vi "main.vi"() -> ()   [LabVIEW 2021]
uses:
  <vilib>/MakerHub/LINX/Private/Device/Type Defs/Stimulus Pulse.ctl
  <vilib>/MakerHub/LINX/Public/Utilities/Open Serial.vi
  <vilib>/MakerHub/LINX/LMH-LINX.lvlib
  <vilib>/MakerHub/LINX/Private/Device/Device.lvlib
panel:
  in  "Knob":dbl(knob) scale=0.0..100.0
  in  "Stop":bool
  out "Error Out":errorcluster
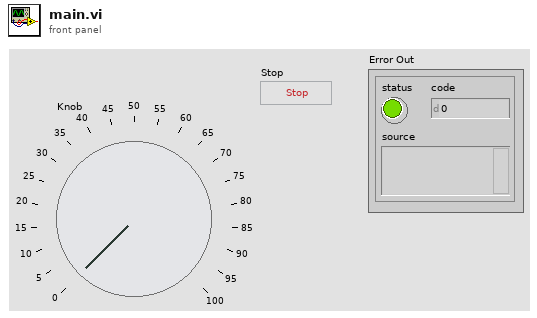
[diagram p1: front panel]
types:
  T1 = typedef "LMH-LINX.lvlib/LINX Ref.ctl" = cluster{"IO":T2, "Interface":T3, "LINX Device Config":T4}
  T2 = typedef "LMH-LINX.lvlib/Platform.ctl" = enum16{"Remote", "Local"}
  T3 = typedef "LMH-LINX.lvlib/Interface.ctl" = enum16{"Serial", "TCP"}
  T4 = typedef "LMH-LINX.lvlib/Device.lvlib/LINX Device Config.ctl" = cluster{"Interface":T3, "COM Port":refnum<visa-resource-name>, "TCP Configuration":T5, "Device Family":u8, "Device ID":u8, "Device Name":string, "TCP Ref":refnum<k5>, "Channels":T6}
  T5 = typedef "LMH-LINX.lvlib/Device.lvlib/TCP Config.ctl" = cluster{"IP Address":string, "Port":u16}
  T6 = typedef "LMH-LINX.lvlib/Channels.ctl" = cluster{"DI":u8[], "DO":u8[], "AI":u8[], "AO":u8[], "PWM":u8[], "QE":u8[], "UART":u8[], "I2C 2":u8[], "SPI":u8[], "CAN":u8[], "Servo":u8[], "AI Ref (V)":dbl, "AI Resolution (Bits)":u8, "AO Ref (V)":dbl, "AO Resolution (Bits)":u8}
  T7 = typedef "LMH-LINX.lvlib/Device.lvlib/Stimulus Pulse.ctl" = enum16{"None", "Active Low", "Active High"}
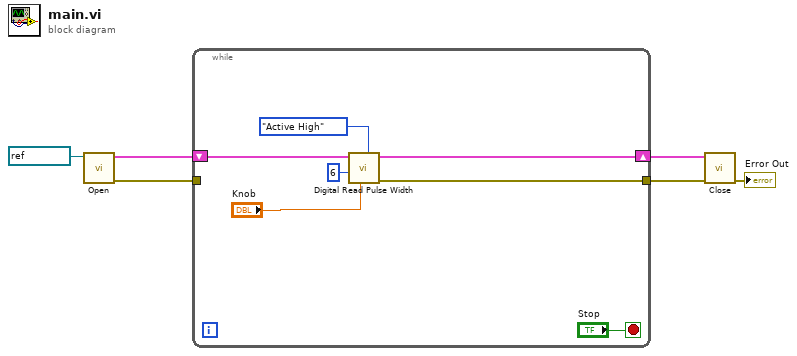
[diagram p0: block diagram]
diagram:
  n1 = call-poly <vilib>:"Open.vi"("Serial Port"=refnum<visa-resource-name> "COM5") -> ("Error Out"=w3:errorcluster, "LINX Resource"=w4:T1)  [unwired: 8 in, 1 out]
  n2 = while {
    tunnel: w3 -> [_]
    shift-right: [w9] -> w1
    shift-left: w4 -> [w12]
    tunnel: [w8] -> w2
    stop <- "Stop" stop-if-true
    n3 = call <vilib>:"Digital Read Pulse Width.vi"("Stimulus Pulse (Active High)"=Stimulus_Pulse."Active High", "Timeout  (250 mS)"="Knob", "DO Channel"=u8 6, "LINX Resource"=w12) -> ("Error Out"=w8:errorcluster, "LINX Resource"=w9:T1)  [unwired: 5 in, 1 out]
  }
  n4 = call <vilib>:"Close.vi"("Error In"=w2, "LINX Resource"=w1) -> ("Error Out"=→"Error Out":errorcluster)  [unwired: 9 in]
